vi "ILCOutputsView.vi"(10 "UserEvents in":refnum<class "UserEvents.lvclass">) -> ()   [LabVIEW 2015, in "FAMTViews.lvlib"]
uses:
  FAMTViews.lvlib
  Typedefs/ADC Outputs.ctl
  UserEvents/UserEvents.lvclass
  UserEvents/UserEvents.lvclass/UserEvents.ctl
  Typedefs/StateSelector.ctl
  Typedefs/FAMTTypedefs.lvlib
panel:
  out "Output Data":T1
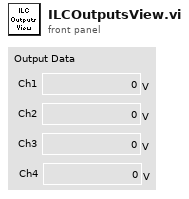
[diagram p1: front panel]
types:
  T1 = typedef "FAMTTypedefs.lvlib/ADC Outputs.ctl" = cluster{"Ch1":dbl[unit], "Ch2":dbl[unit], "Ch3":dbl[unit], "Ch4":dbl[unit]}
  T2 = typedef "FAMTTypedefs.lvlib/PubDataEvents.ctl" = cluster{"State":refnum<user-event>, "ErrorCode":refnum<user-event>, "ADC Outputs":refnum<user-event>, "InputData":refnum<user-event>, "ControllerData":refnum<user-event>, "TestStatus":refnum<user-event>, "LogPath":refnum<user-event>}
  T3 = cluster{"Event Registration Refnum":refnum<event-registration>, "Event Registration Refnum":refnum<event-registration>}
  T4 = typedef "FAMTTypedefs.lvlib/StateSelector.ctl" = enum16{"OfflineState", "FaultState", "StandbyState", "DisabledState", "EnabledState", "WaitForUserInputState", "PerformOpenLoopScanState"}
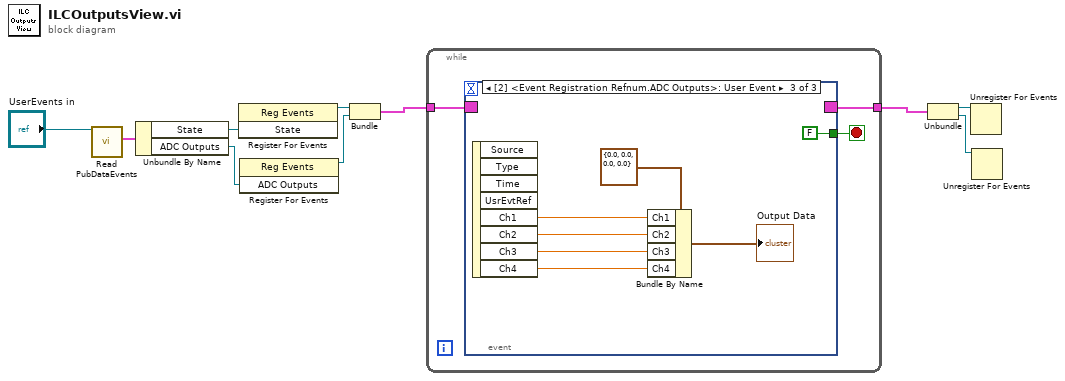
[diagram p0: block diagram]
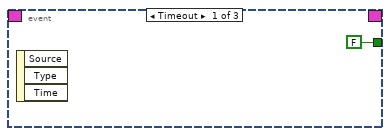
[diagram p2: hidden frame]
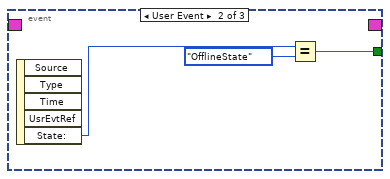
[diagram p3: hidden frame]
diagram:
  n1 = call "Read PubDataEvents.vi"("UserEvents in"="UserEvents in") -> ("PubDataEvents"=w8:T2)  [unwired: 9 in, 1 out]
  n2 = Unbundle By Name(w8) -> ("State"=w9:refnum<user-event>, "ADC Outputs"=w3:refnum<user-event>)
  n3 = register-events(w9) -> (reference out=w10:refnum<event-registration>)  [unwired: 2 in, 1 out]
  n4 = register-events(w3) -> (reference out=w2:refnum<event-registration>)  [unwired: 2 in, 1 out]
  n5 = Bundle("Event Registration Refnum"=w10, "Event Registration Refnum"=w2) -> (w6:T3)  [unwired: 1 in]
  n6 = while {
    tunnel: w6 -> [w13]
    tunnel: [w12] -> w4
    stop <- w11 stop-if-true
    n7 = event shown="[2] <Event Registration Refnum.ADC Outputs>: User Event" {
      selector: w13 -> [_ _ _]
      dyn-events: [_ _ _] -> w12
      timeout: _ -> [_ _ _]
      tunnel: [FALSE w15 FALSE] -> w11
      event Timeout {
        n8 = event-data() -> ()  [unwired: 1 in, 3 out]
      }
      event User Event {
        n9 = event-data() -> ("State:"=w17:T4)  [unwired: 1 in, 4 out]
        n10 = Equal?(x=w17, y=StateSelector."OfflineState") -> (x = y?=w15:bool)
      }
      event User Event {
        n11 = event-data() -> ("Ch1"=w19:dbl[unit], "Ch2"=w20:dbl[unit], "Ch3"=w21:dbl[unit], "Ch4"=w22:dbl[unit])  [unwired: 1 in, 4 out]
        n12 = Bundle By Name(cluster=T1 {"Ch1"=0.0, "Ch2"=0.0, "Ch3"=0.0, "Ch4"=0.0} ("Output Data"), "Ch1"=w19, "Ch2"=w20, "Ch3"=w21, "Ch4"=w22) -> (→"Output Data":T1)
      }
    }
  }
  n13 = Unbundle(w4) -> ("Event Registration Refnum"=w5:refnum<event-registration>, "Event Registration Refnum"=w1:refnum<event-registration>)
  n14 = Unregister For Events(event registration refnum=w5) -> ()  [unwired: 1 in, 1 out]
  n15 = Unregister For Events(event registration refnum=w1) -> ()  [unwired: 1 in, 1 out]
